vi "Main_23A.vi"() -> ()   [LabVIEW 2024]
uses:
  <vilib>/Utility/miscctls.llb/LVMapReplaceAction.ctl
  <vilib>/Utility/error.llb/Trim Whitespace One-Sided.vi
  Utility/Universal Utility/TypeDefs_Utility/Cluster_Row-Column.ctl
  9e3f57c0-2ef8-4495-8287-c6a42a5fb955.vi
  Utility/Universal Utility/TypeDefs_Utility/ENUM_4 Directions U-D-L-R.ctl
  Utility/Universal Utility/TypeDefs_Utility/ENUM_8 Directions U-D-L-R.ctl
panel:
  out "Map":map{string, set{string}}(c390)
  in  "Select Data":enum32{"Example", "Puzzle"}(tab)
  in  "Example":string="kh-tc\nqp-kh\nde-cg\nka-co\nyn-aq\nqp-ub\ncg-tb\nvc-aq\ntb-ka\nwh-tc\nyn-cg\nkh-ub\nta-co\nde-co\ntc-td\ntb-wq\nwh-td\nta-ka\ntd-qp\naq-cg\nwq-ub\nub-vc\nde-ta\nwq-aq\nwq-vc\nwh-yn\nka-de\nkh-ta\nco-tc\nwh-qp\ntb-vc\ntd-yn"
  in  "Puzzle":string="pt-af\nag-sn\nea-le\nhf-iv\nin-sm\nxw-av\nzf-fm\nxl-hj\nqp-hy\njz-rg\nky-iu\ndf-ub\ntq-kh\nel-fr\nqv-pj\nkl-xh\nqg-vf\nri-xm\nlq-yh\nfj-al\nka-so\ncm-qk\nxt-eo\nje-do\nlj-lb\njz-sv\ngw-th\ndo-dn\npy-jb\nmx-hq\nnb-jx\nkg-ca\naa-mc\nhn-ra\nik-iu\nvn-tn\njr-jv\npc-ph\nog-eg\nkj-oj\nmu-xn\nei-ad\nwg-jl\nzv-ma\nyz-qn\nrr-qq\npk-sc\nnf-ne\nue-dx\npw-pb\nds-gw\nfl-xt\nhk-lm\nil-ec\nbf-qt\nhu-ph\nnu-fq\nit-jy\npt-mp\nwu-fw\neu-aq\npr-hf\nnb-ia\nmx-kd\nlj-ed\njr-zs\nxv-mv\nad-iq\npq-wx\nir-ix\nfa-xy\nzb-jn\nla-kk\nqb-ni\nze-gn\nlk-ar\nkw-fl\nsp-sa\nns-ka\ncx-ag\nic-rx\nkx-jb\njn-fp\noq-tp\ntt-zn\nqk-rj\nus-ww\ney-nx\njf-gi\npj-ko\nvp-ix\nfs-el\nav-rg\nsc-ey\nwt-tm\nra-ol\nqm-mo\nll-bf\nxf-yz\nzz-he\n..."
  out "Answer 1062":u32
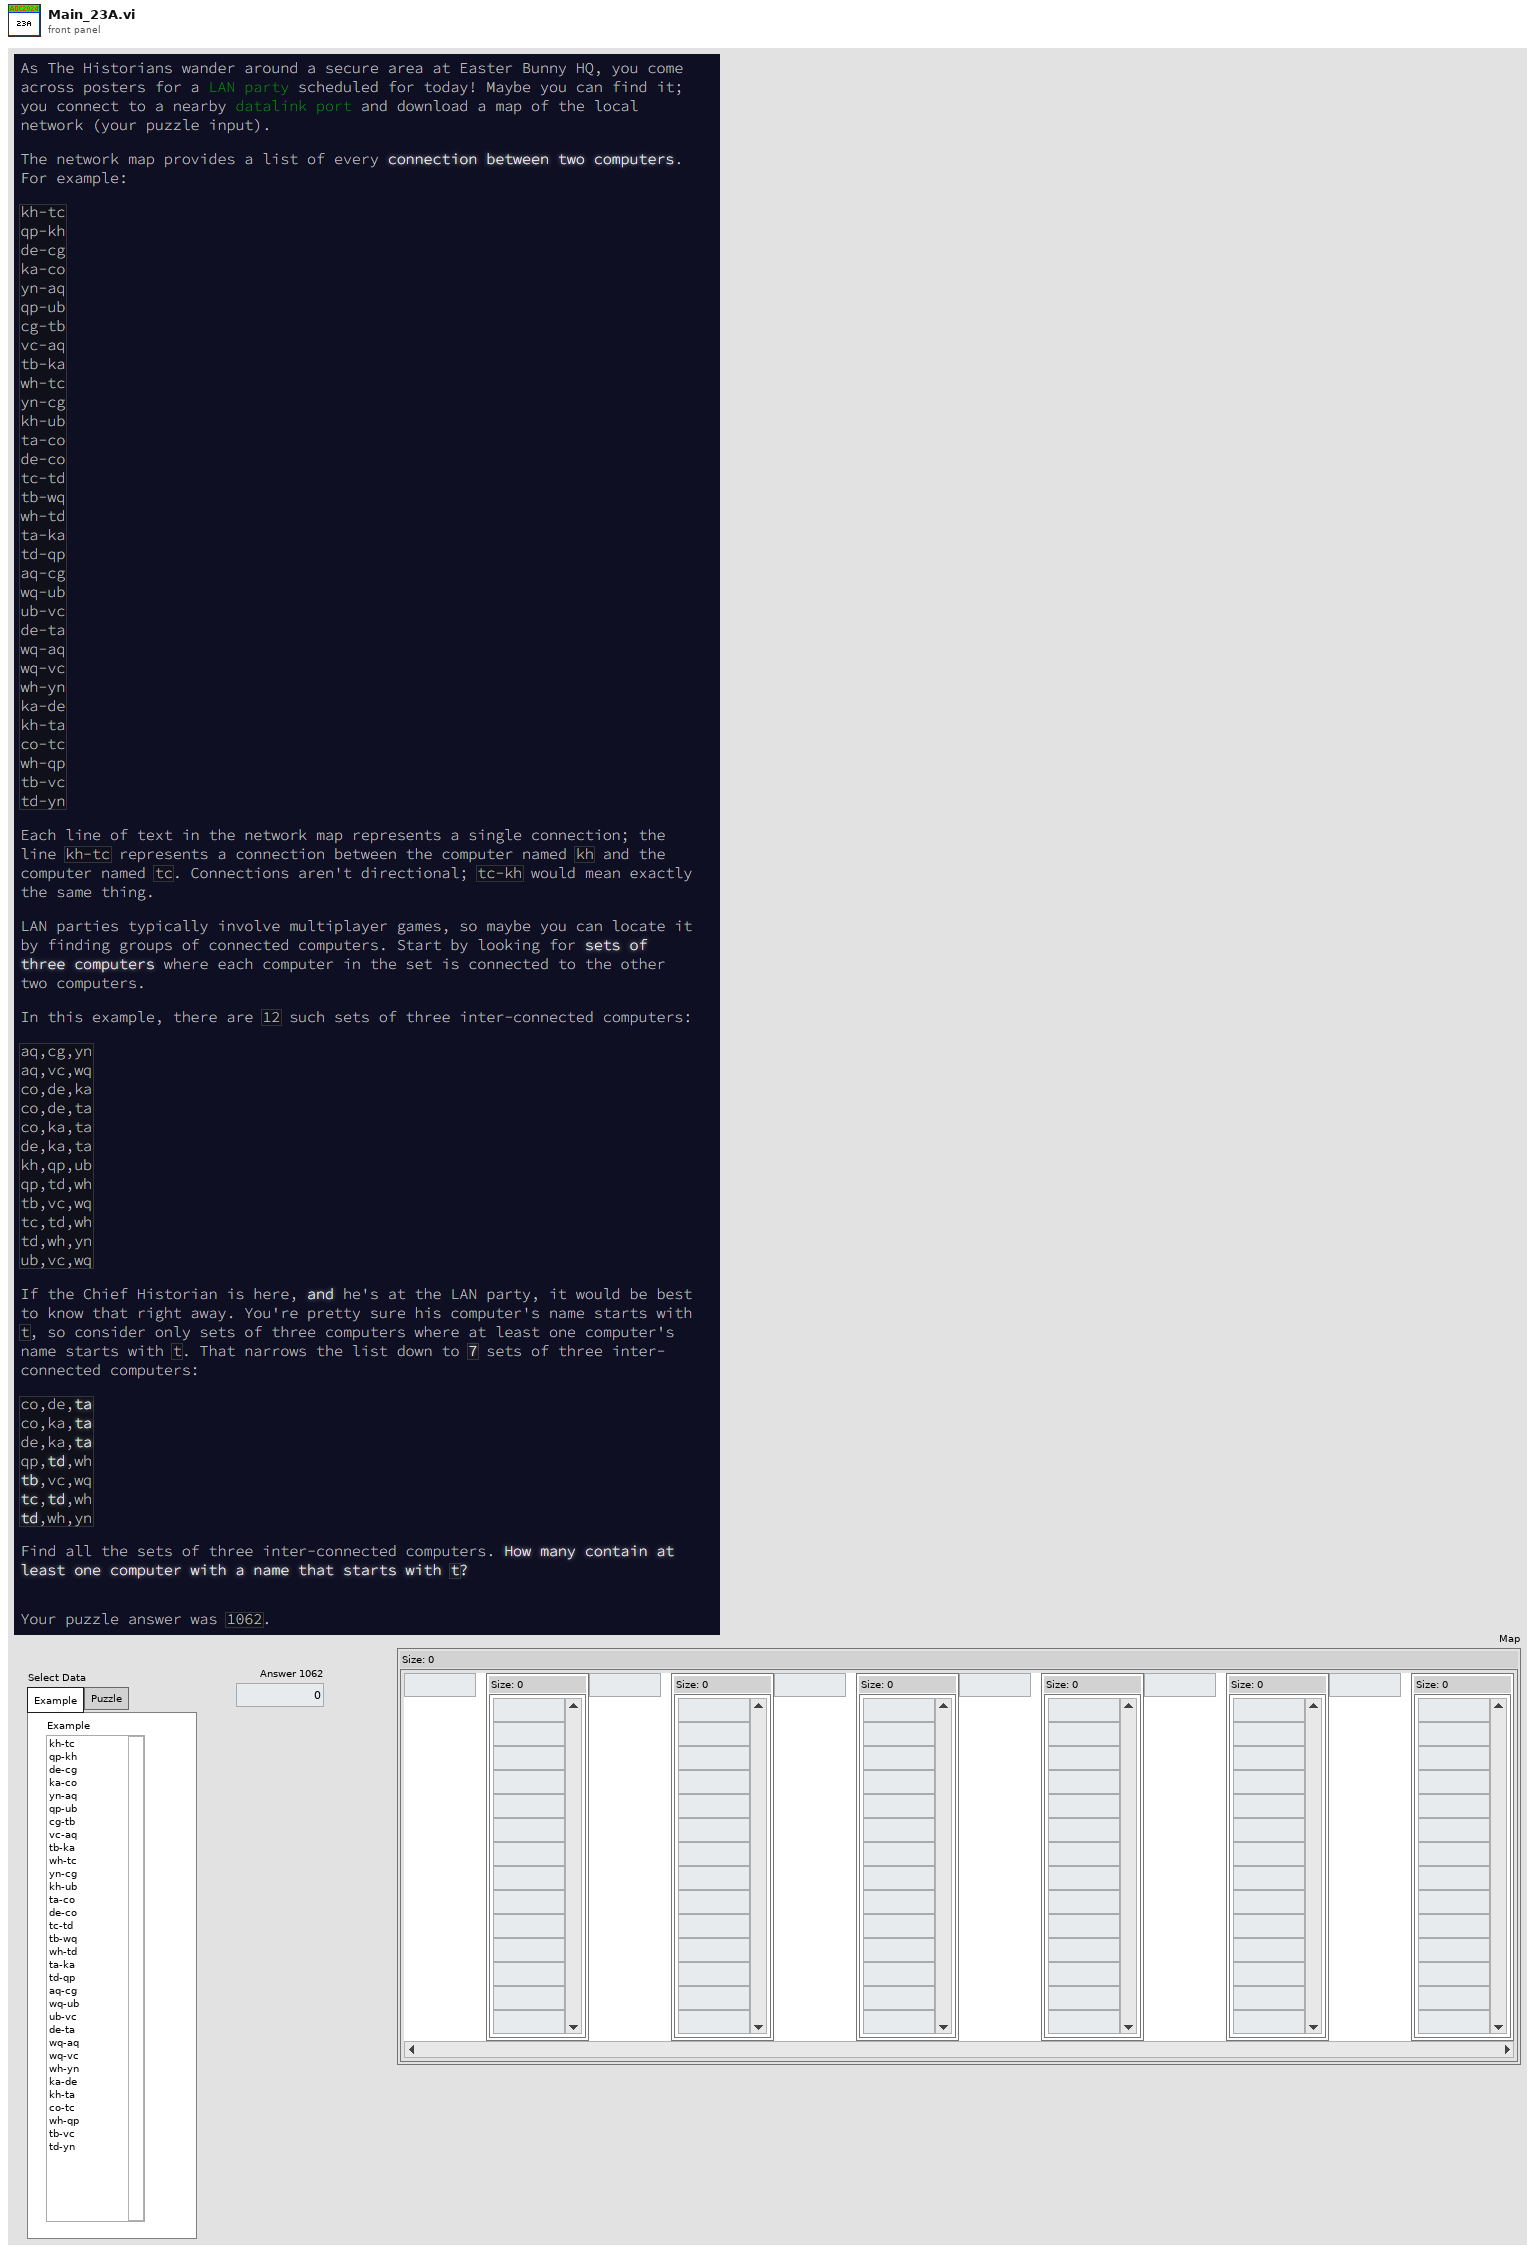
[diagram p1: front panel]
types:
  T1 = typedef "ENUM_8 Directions U-D-L-R.ctl" = enum16{"Up;-1,0", "Up-Right;-1,1", "Right;0,1", "Down-Right;1,1", "Down;1,0", "Down-Left;1,-1", "Left;0,-1", "Up-Left;-1,-1"}
  T2 = typedef "ENUM_4 Directions U-D-L-R.ctl" = enum16{"Up;-1,0", "Right;0,1", "Down;1,0", "Left;0,-1"}
  T3 = typedef "Cluster_Row-Column.ctl" = cluster{"R":i32, "C":i32}
  T4 = typedef "LVMapReplaceAction.ctl" = enum32{"Modify Entry only if found", "Add or Modify Entry", "Delete Entry"}
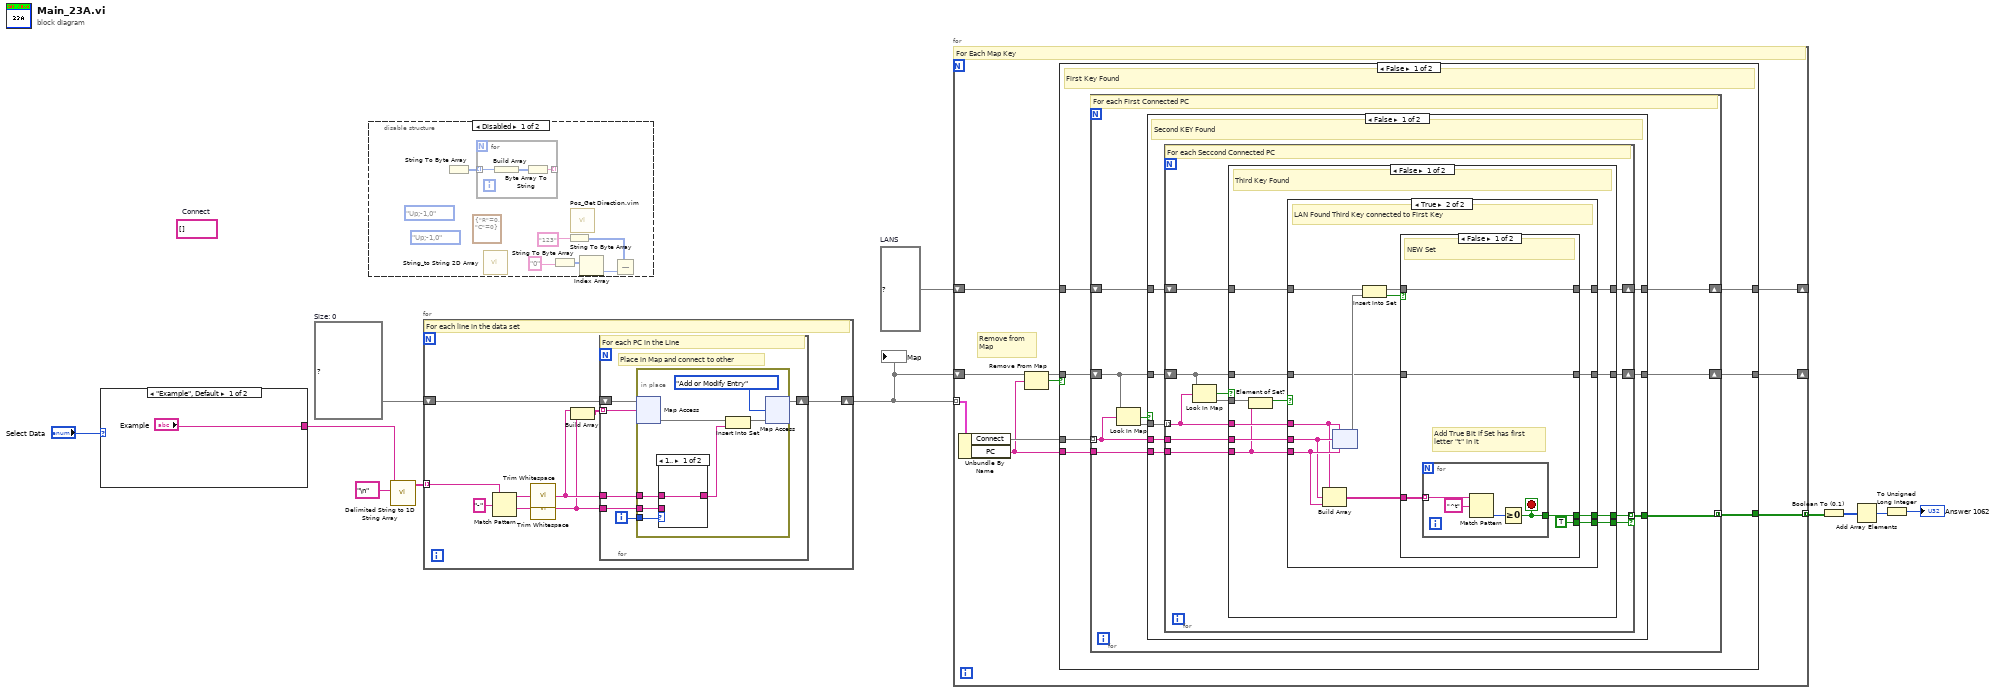
[diagram p0: block diagram]
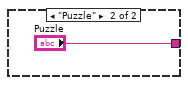
[diagram p7: hidden frame]
diagram:
  w1 = set{set{string}} {}  # LANS
  (unwired) string[] []  # Connect
  w6 = map{string, set{string}} {}  # Size: 0
  n1 = case shown="\"Example\", Default" "Select Data" {
    tunnel: ["Example" "Puzzle"] -> w7
    frame "Example", Default {
    }
    frame "Puzzle" {
    }
  }
  n2 = disable-structure shown="Disabled" {
    frame Disabled {
      (unwired) ENUM_8_Directions_U-D-L-R."Up;-1,0" ("Direction 8")
      (unwired) ENUM_4_Directions_U-D-L-R."Up;-1,0" ("Direction")
      (unwired) T3 {"R"=0, "C"=0} ("Position")
      n3 = String To Byte Array() -> (unsigned byte array=w14:u8[])  [unwired: 1 in]
      n4 = for {
        tunnel: w14 -> [w22] mode=indexing
        tunnel: [w20] -> _ mode=indexing
        n5 = Build Array(w22) -> (w21:u8[])
        n6 = Byte Array To String(unsigned byte array=w21) -> (string=w20:string)
      }
      n7 = call "String_to String 2D Array.vi"() -> ()  [unwired: 11 in, 1 out]
      n8 = String To Byte Array(string="0") -> (unsigned byte array=w17:u8[])
      n9 = String To Byte Array(string="123") -> (unsigned byte array=w15:u8[])
      n10 = call "Pos_Get Direction.vim"() -> ()  [unwired: 11 in, 1 out]
      n11 = Index Array(array=w17) -> (element=w16:u8)  [unwired: 1 in]
      n12 = Subtract(x=w15, y=w16) -> ()  [unwired: 1 out]
    }
    frame Enabled {
    }
  }
  n13 = call <vilib>:"Delimited String to 1D String Array.vi"("delimiter"="\n" ("delimiter (Tab)"), "delimited string"=w7) -> ("string array"=w10:string[])  [unwired: 9 in]
  n14 = for {
    tunnel: w10 -> [w31] mode=indexing
    shift-right: [w26] -> w5
    shift-left: w6 -> [w27]
    # "For each line in the data set"
    n15 = Match Pattern(string=w31, regular expression="-") -> (before substring=w29:string, after substring=w28:string)  [unwired: 1 in, 2 out]
    n16 = call <vilib>:"Trim Whitespace.vi"("string"=w29) -> ("trimmed string"=w24:string)  [unwired: 1 in]
    n17 = call <vilib>:"Trim Whitespace.vi"("string"=w28) -> ("trimmed string"=w23:string)  [unwired: 1 in]
    n18 = Build Array(w24, w23) -> (w25:string[])
    n19 = for {
      shift-right: [w36] -> w26
      shift-left: w27 -> [w37]
      tunnel: w25 -> [w35] mode=indexing
      tunnel: w24 -> [w32]
      tunnel: w23 -> [w33]
      i -> [w34]
      # "Place in Map and connect to other"
      # "For each PC in the Line"
      n20 = in-place {
        in-place-border: w34 -> [w43]
        in-place-border: w33 -> [w42]
        in-place-border: w32 -> [w41]
        n21 = in-place-map #1(w37, w35) -> (w40:set{string})  [unwired: 1 in, 1 out]
        n22 = case shown="1.." w43 {
          tunnel: w42 -> [_ w46]
          tunnel: w41 -> [w45 _]
          tunnel: [w45 w46] -> w38
          frame 1.. {
          }
          frame ..0 {
          }
        }
        n23 = Insert Into Set(10:w38, 11:w40) -> (3:w39:set{string})  [unwired: 1 out]
        n24 = in-place-map #1(w39, LVMapReplaceAction."Add or Modify Entry" ("action")) -> (w36:map{string, set{string}})  [unwired: 2 out]
      }
    }
  }
  "Map" <- w5
  n25 = for {
    tunnel: w5 -> [w56] mode=indexing
    tunnel: [w54] -> w4 mode=concatenating
    shift-right: [w52] -> _
    shift-left: w1 -> [w53]
    shift-right: [w51] -> _
    shift-left: w5 -> [w48]
    # "Remove from\nMap"
    # "For Each Map Key"
    n26 = Unbundle By Name(w56) -> ("Connect"=w55:set{string}, "PC"=w50:string)
    n27 = Remove From Map(10:w50, 11:w48) -> (2:w49:bool, 3:w47:map{string, set{string}})  [unwired: 1 out]
    n28 = case shown="False" w49 {
      tunnel: w55 -> [w63 _]
      tunnel: [w62 _] -> w54
      tunnel: w53 -> [w61 w134]
      tunnel: [w60 w134] -> w52
      tunnel: [w59 w133] -> w51
      tunnel: w47 -> [w58 w133]
      tunnel: w50 -> [w57 _]
      frame False {
        # "First Key Found"
        n29 = for {
          tunnel: w63 -> [w69] mode=indexing
          tunnel: w57 -> [w70]
          tunnel: [w68] -> w62 mode=concatenating
          shift-right: [w66] -> w60
          shift-left: w61 -> [w67]
          shift-right: [w65] -> w59
          shift-left: w58 -> [w71]
          # "For each First Connected PC"
          n30 = Look In Map(map=w71, key=w69) -> (key not found?=w64:bool, value=w72:set{string})  [unwired: 1 in]
          n31 = case shown="False" w64 {
            tunnel: w72 -> [w80 _]
            tunnel: w71 -> [w79 w131]
            tunnel: w70 -> [w78 _]
            tunnel: w69 -> [w77 _]
            tunnel: [w76 _] -> w68
            tunnel: w67 -> [w75 w132]
            tunnel: [w74 w132] -> w66
            tunnel: [w73 w131] -> w65
            frame False {
              # "Second KEY Found"
              n32 = for {
                tunnel: w80 -> [w90] mode=indexing
                tunnel: w78 -> [w88]
                tunnel: w77 -> [w89]
                tunnel: [w87] -> w76 mode=indexing if=w82
                shift-right: [w85] -> w74
                shift-left: w75 -> [w86]
                shift-right: [w83] -> w73
                shift-left: w79 -> [w84]
                # "For each Seccond Connected PC"
                n33 = Look In Map(map=w84, key=w90) -> (key not found?=w81:bool, value=w91:set{string})  [unwired: 1 in]
                n34 = case shown="False" w81 {
                  tunnel: w91 -> [w102 _]
                  tunnel: w90 -> [w101 _]
                  tunnel: w89 -> [w100 _]
                  tunnel: w88 -> [w99 _]
                  tunnel: [w98 _] -> w87
                  tunnel: w86 -> [w96 w130]
                  tunnel: [w95 w130] -> w85
                  tunnel: w84 -> [w94 w129]
                  tunnel: [w93 w129] -> w83
                  tunnel: [w92 _] -> w82
                  frame False {
                    # "Third Key Found"
                    n35 = Element of Set?(10:w99, 11:w102) -> (3:w97:bool)
                    n36 = case shown="True" w97 {
                      tunnel: w101 -> [_ w113]
                      tunnel: w100 -> [_ w114]
                      tunnel: w99 -> [_ w115]
                      tunnel: [_ w116] -> w98
                      tunnel: w96 -> [w104 w112]
                      tunnel: [w104 w108] -> w95
                      tunnel: w94 -> [w103 w107]
                      tunnel: [w103 w106] -> w93
                      tunnel: [_ w105] -> w92
                      frame False {
                        # "No LAN"
                      }
                      frame True {
                        # "LAN Found Third Key connected to First Key"
                        n37 = Build Array(w113, w114, w115) -> (w117:string[])
                        n38 = node(w113, w114, w115) -> (w111:set{string})
                        n39 = Insert Into Set(10:w111, 11:w112) -> (2:w110:bool, 3:w109:set{set{string}})
                        n40 = case shown="False" w110 {
                          tunnel: w117 -> [w122 _]
                          tunnel: [w121 _] -> w116
                          tunnel: w109 -> [w120 w128]
                          tunnel: [w120 w128] -> w108
                          tunnel: w107 -> [w118 w127]
                          tunnel: [w118 w127] -> w106
                          tunnel: [TRUE _] -> w105
                          frame False {
                            # "Add True Bit if Set has first \nletter \"t\" in it"
                            # "NEW Set"
                            n41 = for {
                              tunnel: w122 -> [w123] mode=indexing
                              tunnel: [w124] -> w121
                              stop <- w124 stop-if-true
                              n42 = Match Pattern(string=w123, regular expression="^t") -> (offset past match=w125:i32)  [unwired: 1 in, 3 out]
                              n43 = Greater Or Equal To 0?(x=w125) -> (x >= 0?=w124:bool)
                            }
                          }
                          frame True {
                            # "Already Found this Set"
                          }
                        }
                      }
                    }
                  }
                  frame True {
                    # "Third Key Removed"
                  }
                }
              }
            }
            frame True {
              # "Second Key Removed"
            }
          }
        }
      }
      frame True {
        # "First Key Removed"
      }
    }
  }
  n44 = Boolean To (0,1)(Boolean=w4) -> (0, 1=w3:i16[])
  n45 = Add Array Elements(numeric array=w3) -> (sum=w2:i16)
  n46 = To Unsigned Long Integer(number=w2) -> (unsigned 32bit integer=→"Answer 1062":u32)
